vi "Write Value.vi"(8 "error in (no error)":errorcluster, 10 "Value":bool, 11 "bt_Blackboard Boolean Set in":refnum<class "bt_Blackboard Boolean Set.lvclass">) -> (0 "error out":errorcluster, 3 "bt_Blackboard Boolean Set out":refnum<class "bt_Blackboard Boolean Set.lvclass">)   [LabVIEW 2021, in "BT.lvlib" / "bt_Blackboard Boolean Set.lvclass"]
uses:
  bt_Blackboard Boolean Set.lvclass
  bt_Blackboard Boolean Set.lvclass/bt_Blackboard Boolean Set.ctl
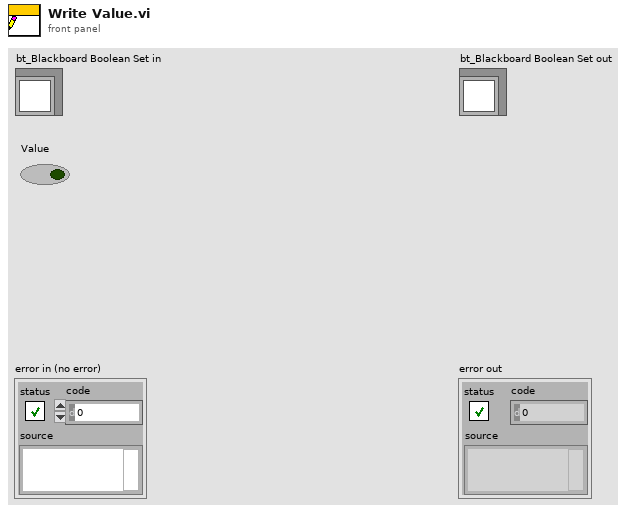
[diagram p1: front panel]
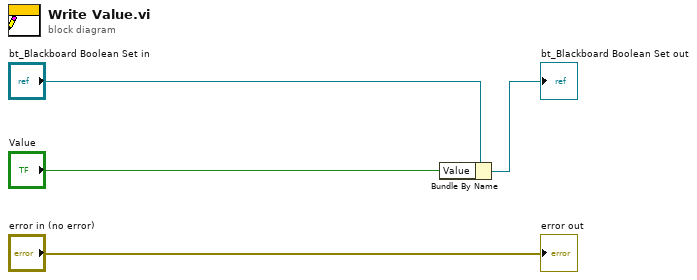
[diagram p0: block diagram]
diagram:
  n1 = Bundle By Name(cluster="bt_Blackboard Boolean Set in", "Value"="Value") -> (→"bt_Blackboard Boolean Set out":refnum<class "bt_Blackboard Boolean Set.lvclass">)
  "error out" <- "error in (no error)"
